vi "InitializeGlobalVariables.vi"(11 "TSM Context":T1) -> (0 "error out":errorcluster)   [LabVIEW 2019]
uses:
  <vilib>/NI_TestStand_SemiconductorModule/NI_TestStand_Semiconductor_Module.lvlibp/PinMap/General/SemiconductorModuleContext.ctl
  TSM Context Data Access/TSM Context Data Access.lvclass/TSM Context Data Access.ctl
  TSM Context Data Access/Public/Properties/A - Write.vi
  <vilib>/NI_TestStand_SemiconductorModule/NI_TestStand_Semiconductor_Module.lvlibp/PinMap/Site and Global Data/SetSiteData.vi
  TSM Context Data Access/TSM Context Data Access.lvclass
  <vilib>/NI_TestStand_SemiconductorModule/NI_TestStand_Semiconductor_Module.lvlibp
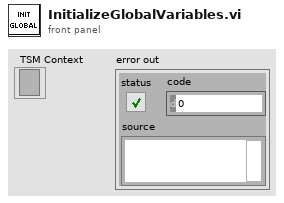
[diagram p1: front panel]
types:
  T1 = typedef "NI_TestStand_Semiconductor_Module.lvlibp/SemiconductorModuleContext.ctl" = refnum<k7>
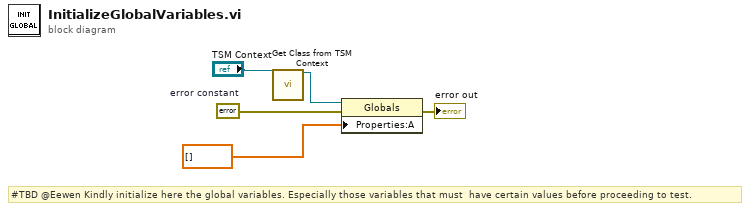
[diagram p0: block diagram]
diagram:
  w3 = errorcluster {"status"=FALSE, "code"=0, "source"=""}  # error constant
  # "#TBD @Eewen Kindly initialize here the global variables. Especially those variables that must  have certain values before proceeding to test."
  n1 = call "Get Class from TSM Context.vi"("TSM Context"="TSM Context") -> ("Global Memory Class"=w4:refnum<class "TSM Context Data Access.lvclass">)  [unwired: 14 in]
  n2 = property class="Globals"(reference=w4, error in=w3, "Properties:A"=dbl[] [] ("A")) -> (error out=→"error out":errorcluster)  [unwired: 1 out]
